vi "Configure Operation Mode.vi"(8 "error in (no error)":errorcluster, 9 "Range (15.00)":dbl=15.0001 min=0.0001 max=500.0 step=1.0 format="%.2f", 10 "Operation Mode (0:CC)":u16(ring) items=["CC", "CV", "CR", "CW"], 11 "VISA resource name":refnum<visa-resource-name>) -> (0 "error out":errorcluster, 3 "VISA resource name out":refnum<visa-resource-name>)   [LabVIEW 2024, in "BK Precision 8500B Series.lvlib"]
doc: "Configures the operation mode, range (for CC and CV mode)."
uses:
  BK Precision 8500B Series.lvlib
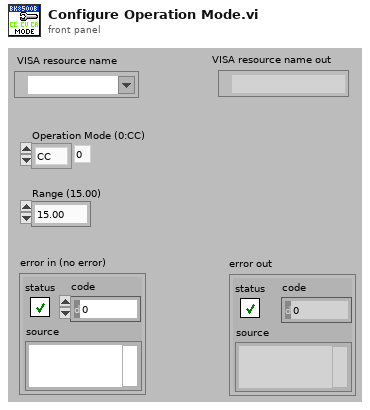
[diagram p1: front panel]
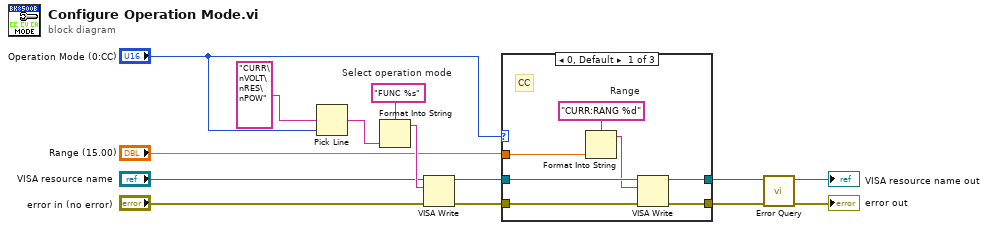
[diagram p0: block diagram]
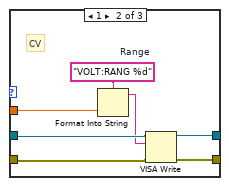
[diagram p2: hidden frame]
diagram:
  w12 = "FUNC %s"  # Select operation mode
  n1 = Pick Line(multi-line string="CURR\nVOLT\nRES\nPOW", line index="Operation Mode (0:CC)") -> (output string=w9:string)  [unwired: 1 in]
  n2 = Format Into String(format string=w12, w9) -> (resulting string=w11:string)  [unwired: 2 in, 1 out]
  n3 = VISA Write(VISA resource name="VISA resource name", write buffer=w11, error in (no error)="error in (no error)") -> (VISA resource name out=w6:refnum<visa-resource-name>, error out=w7:errorcluster)  [unwired: 1 out]
  n4 = case shown="0, Default" "Operation Mode (0:CC)" {
    tunnel: w7 -> [w16 w24 w29]
    tunnel: w6 -> [w17 w23 w30]
    tunnel: [w21 w28 w30] -> w5
    tunnel: [w20 w27 w29] -> w4
    tunnel: "Range (15.00)" -> [w18 w25 _]
    frame 0, Default {
      w19 = "CURR:RANG %d"  # Range
      # "CC"
      n5 = Format Into String(format string=w19, w18) -> (resulting string=w15:string)  [unwired: 2 in, 1 out]
      n6 = VISA Write(VISA resource name=w17, write buffer=w15, error in (no error)=w16) -> (VISA resource name out=w21:refnum<visa-resource-name>, error out=w20:errorcluster)  [unwired: 1 out]
    }
    frame 1 {
      w26 = "VOLT:RANG %d"  # Range
      # "CV"
      n7 = Format Into String(format string=w26, w25) -> (resulting string=w22:string)  [unwired: 2 in, 1 out]
      n8 = VISA Write(VISA resource name=w23, write buffer=w22, error in (no error)=w24) -> (VISA resource name out=w28:refnum<visa-resource-name>, error out=w27:errorcluster)  [unwired: 1 out]
    }
    frame 2, 3 {
      # "CW"
      # "CR"
    }
  }
  n9 = call "Error Query.vi"("error in (no error)"=w4, "VISA resource name"=w5) -> ("error out"=→"error out":errorcluster, "VISA resource name out"=→"VISA resource name out":refnum<visa-resource-name>)  [unwired: 6 in, 2 out]
